vi "A3_cmd.reply.vi"(8 "error in":errorcluster, 10 "cmd":string, 11 "VISA resource name":refnum<visa-resource-name>="COM6") -> (0 "error out":errorcluster, 2 "reply":string, 3 "VISA resource name out":refnum<visa-resource-name>)   [LabVIEW 2022 SP3]
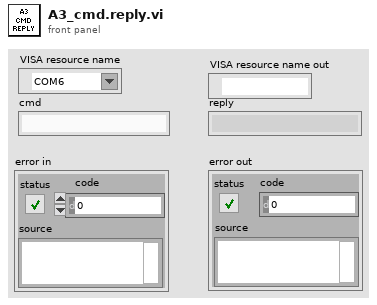
[diagram p1: front panel]
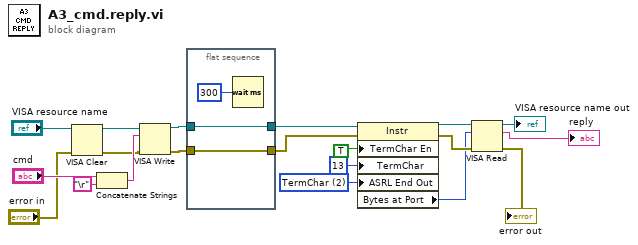
[diagram p0: block diagram]
diagram:
  w8 = u16 2 items=["None", "Last Bit", "TermChar", "Break"] ("Serial Settings:End Mode for Writes")
  n1 = VISA Clear(VISA resource name="VISA resource name", error in (no error)="error in") -> (VISA resource name out=w17:refnum<visa-resource-name>, error out=w1:errorcluster)
  n2 = Concatenate Strings("cmd", "\r") -> (w11:string)
  n3 = VISA Write(VISA resource name=w17, write buffer=w11, error in (no error)=w1) -> (VISA resource name out=w6:refnum<visa-resource-name>, error out=w4:errorcluster)  [unwired: 1 out]
  n4 = flat-sequence {
    tunnel: w6 -> [w22]
    tunnel: [w22] -> w5
    tunnel: w4 -> [w21]
    tunnel: [w21] -> w3
    frame #0 {
      n5 = Wait (ms)(milliseconds to wait=u32 300) -> ()  [unwired: 1 out]
    }
  }
  n6 = property class="Instr"(reference=w5, error in=w3, "TermChar En"=TRUE ("Message Based Settings:Termination Character Enable"), "TermChar"=u8 13 ("Message Based Settings:Termination Character"), "ASRL End Out"=w8) -> (reference out=w16:refnum<visa-resource-name>, error out=w13:errorcluster, "Bytes at Port"=w7:u32)
  n7 = VISA Read(VISA resource name=w16, byte count=w7, error in (no error)=w13) -> (VISA resource name out=→"VISA resource name out":refnum<visa-resource-name>, read buffer=→"reply":string, error out=→"error out":errorcluster)  [unwired: 1 out]
